vi "Get Offset Tuning.vi"(8 "error in (no error)":errorcluster, 11 "RTL-SDR in":refnum<class "RTL-SDR.lvclass">) -> (0 "error out":errorcluster, 2 "Enabled?":bool, 3 "RTL-SDR out":refnum<class "RTL-SDR.lvclass">)   [LabVIEW 2015, in "RTL-SDR.lvclass"]
doc: "Created IvanLis by LabVIEW Portal\nProfile: http://labviewportal.org/memberlist.php?mode=viewprofile&u=987\neMail: IvanLisanov@gMail.com\nTelegram: https://t.me/IvanLis"
uses:
  RTL-SDR.lvclass
  RTL-SDR.lvclass/RTL-SDR.ctl
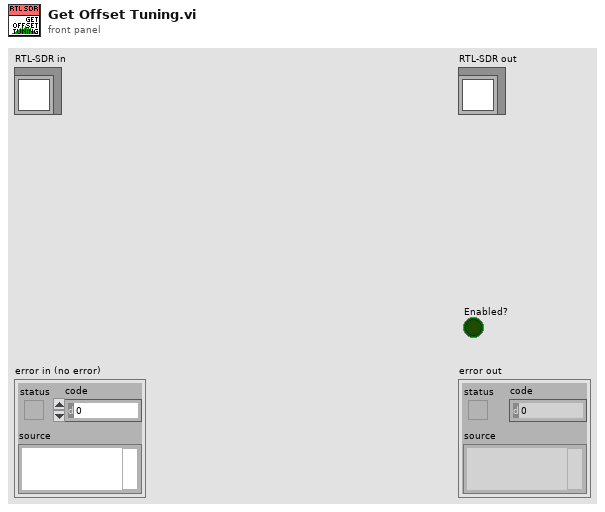
[diagram p1: front panel]
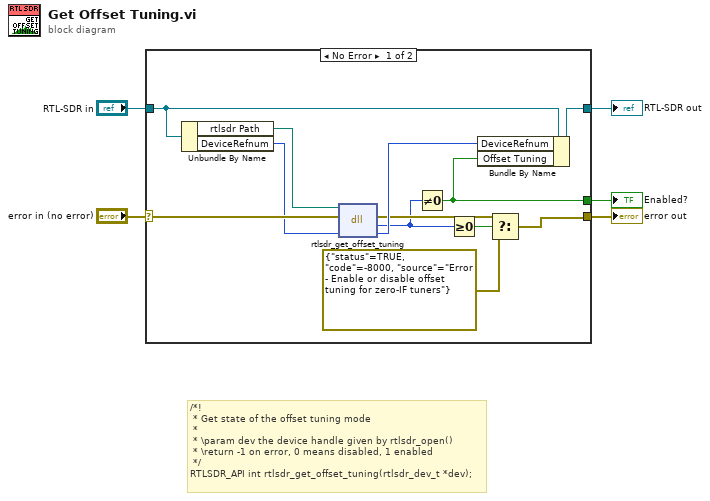
[diagram p0: block diagram]
diagram:
  # "/*!\n * Get state of the offset tuning mode\n *\n * \\param dev the device handle given by rtlsdr_open()\n * \\return -1 on error, 0 means disabled, 1 enabled\n */\nRTLSDR_API int rtlsdr_get_offset_tuning(rtlsdr_dev_t *dev);"
  n1 = case shown="No Error" "error in (no error)" {
    selector: "error in (no error)" -> [w17 w19]
    tunnel: [w7 w19] -> w4
    tunnel: [w13 w18] -> w2
    tunnel: "RTL-SDR in" -> [w16 w18]
    tunnel: [w11 _] -> w1
    frame No Error {
      n2 = Unbundle By Name(w16) -> ("rtlsdr Path"=w15:path, "DeviceRefnum"=w14:u64)
      n3 = dll-call lib="C:/Users/Ivan/Desktop/D-23-09-24 (RTL-SDR)/Project (Pelleng-SDR)/RTL-SDR Class/dll/rtlsdr.*" fn="rtlsdr_get_offset_tuning"(path in=w15, error in=w17, "DeviceRefnum"=w14) -> (error out=w8:errorcluster, "return type"=w6:i32, "DeviceRefnum"=w12:u64)  [unwired: 1 in, 1 out]
      n4 = Not Equal To 0?(x=w6) -> (x != 0?=w11:bool)
      n5 = Greater Or Equal To 0?(x=w6) -> (x >= 0?=w10:bool)
      n6 = Bundle By Name(cluster=w16, "DeviceRefnum"=w12, "Offset Tuning"=w11) -> (w13:refnum<class "RTL-SDR.lvclass">)
      n7 = Select(t=w8, s=w10, f=errorcluster {"status"=TRUE, "code"=-8000, "source"="Error - Enable or disable offset tuning for zero-IF tuners"} ("error out")) -> (s? t:f=w7:errorcluster)
    }
    frame Error {
    }
  }
  "error out" <- w4
  "RTL-SDR out" <- w2
  "Enabled?" <- w1
